vi "ISO8601Timestamp.vi"() -> (0 "ISO8601 Timestamp":string)   [LabVIEW 2013, in "SetListPrefs.lvclass"]
uses:
  SetListPrefs.lvclass
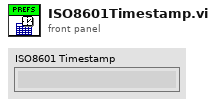
[diagram p1: front panel]
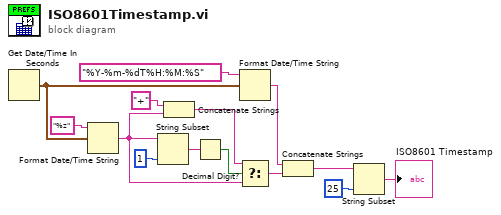
[diagram p0: block diagram]
diagram:
  n1 = Get Date/Time In Seconds() -> (seconds since 1Jan1904=w10:timestamp)
  n2 = Format Date/Time String(time format string (%c)="%z", seconds (now)=w10) -> (date/time string=w4:string)  [unwired: 1 in]
  n3 = String Subset(string=w4, length (rest)=1 ("length (rest)")) -> (substring=w8:string)  [unwired: 1 in]
  n4 = Concatenate Strings("+" ("string"), w4) -> (w5:string)
  n5 = Decimal Digit?(1:w8) -> (0:w6:bool)
  n6 = Format Date/Time String(time format string (%c)="%Y-%m-%dT%H:%M:%S", seconds (now)=w10) -> (date/time string=w3:string)  [unwired: 1 in]
  n7 = Select(t=w5, s=w6, f=w4) -> (s? t:f=w2:string)
  n8 = Concatenate Strings(w3, w2) -> (w1:string)
  n9 = String Subset(string=w1, length (rest)=25 ("length (rest)")) -> (substring=→"ISO8601 Timestamp":string)  [unwired: 1 in]
